vi "burst_frac.vi"(0 "Scale Factor":dbl=1.0, 1 "Upper Pressure":dbl=1.0, 2 "B(x)":dbl[](array[numeric]), 3 "Gs(x)":dbl[][](array[numeric]), 4 "Names":string[](array[string])) -> (5 "Array":cluster{"Ramp Pattern":dbl[], "Array":dbl[]}[](array[cluster]), 6 "Frac Names":string[](array[string]))   [LabVIEW 2013]
uses:
  <vilib>/Analysis/NI_AALPro.lvlib
  <vilib>/Analysis/NI_AALBase.lvlib
  <vilib>/Analysis/1siggen.llb/Ramp Pattern by Delta.vi
  <vilib>/Analysis/polynomials.llb/1D Polynomial Evaluation (DBL).vi
panel:
  out "size(s)":i32
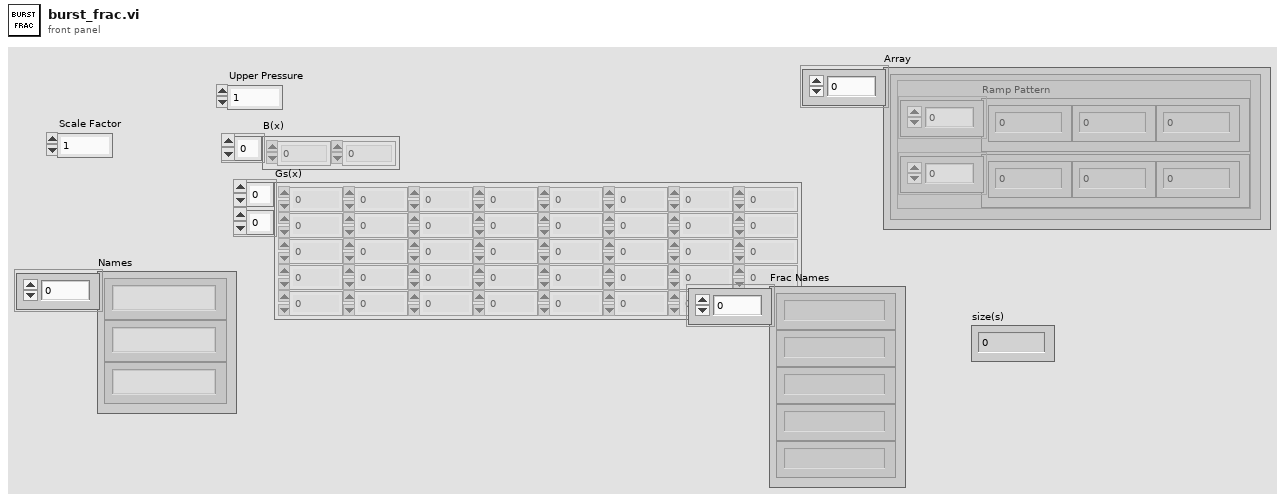
[diagram p1: front panel]
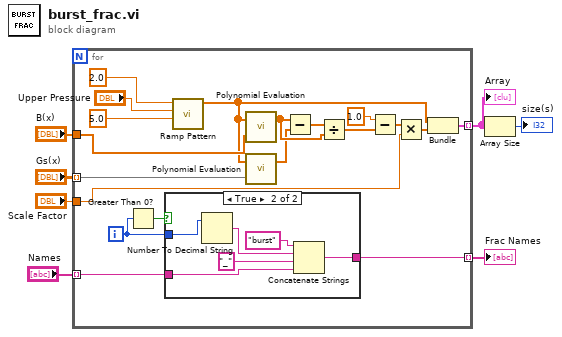
[diagram p0: block diagram]
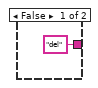
[diagram p2: hidden frame]
diagram:
  n1 = for {
    tunnel: "B(x)" -> [w22]
    tunnel: "Gs(x)" -> [w23] mode=indexing
    tunnel: [w19] -> w3 mode=indexing
    tunnel: [w14] -> w5 mode=indexing
    tunnel: "Names" -> [w13] mode=indexing
    tunnel: "Scale Factor" -> [w8]
    i -> [w11]
    n2 = Greater Than 0?(x=w11) -> (x > 0?=w12:bool)
    n3 = case shown="True" w12 {
      tunnel: w11 -> [_ w33]
      tunnel: ["del" w32] -> w14
      tunnel: w13 -> [_ w28]
      frame False {
      }
      frame True {
        n4 = Number To Decimal String(number=w33) -> (decimal integer string=w30:string)  [unwired: 1 in]
        n5 = Concatenate Strings("burst", w30, "_" ("string"), w28) -> (w32:string)
      }
    }
    n6 = call-poly <vilib>:"Ramp Pattern.vi"("start"=5.0, "end"="Upper Pressure", "delta"=2.0) -> ("Ramp Pattern"=w21:dbl[])  [unwired: 6 in, 2 out]
    n7 = call-poly <vilib>:"Polynomial Evaluation.vi"("P(x)"=w22, "A"=w21) -> ("P(A)"=w20:dbl[])  [unwired: 1 out]
    n8 = call-poly <vilib>:"Polynomial Evaluation.vi"("P(x)"=w23, "A"=w21) -> ("P(A)"=w15:dbl[])  [unwired: 1 out]
    n9 = Subtract(x=w20, y=w15) -> (x-y=w16:dbl[])
    n10 = Divide(x=w16, y=w20) -> (x/y=w18:dbl[])
    n11 = Subtract(x=1.0, y=w18) -> (x-y=w10:dbl[])
    n12 = Multiply(x=w10, y=w8) -> (x*y=w9:dbl[])
    n13 = Bundle("Ramp Pattern"=w21, w9) -> (w19:cluster{"Ramp Pattern":dbl[], dbl[]})  [unwired: 1 in]
  }
  "Array" <- w3
  "Frac Names" <- w5
  n14 = Array Size(array=w3) -> (size(s)=→"size(s)":i32)
